vi "ROI entry-Set ROI tool on Clear All.vi"(8 "error in (no error)":errorcluster, 11 "Last ROI ID Enum":T1) -> (0 "error out":errorcluster)   [LabVIEW 2013]
uses:
  Typedefs/ROI ID Enum.ctl
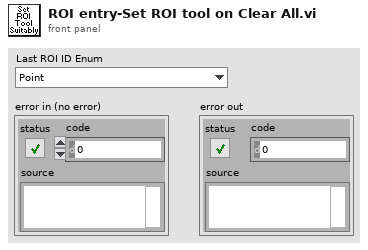
[diagram p1: front panel]
types:
  T1 = typedef "ROI ID Enum.ctl" = enum16{"Point", "MiniScan", "Comp. MiniScan", "Rectangle", "Comp. volume", "Arb. plane point"}
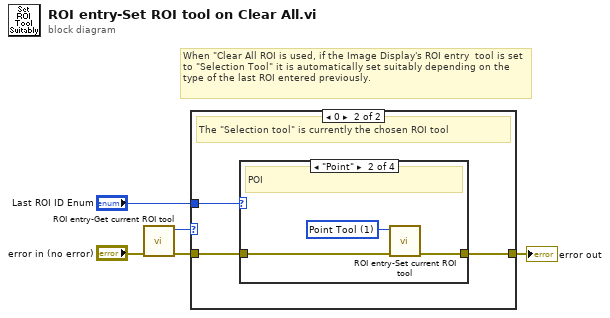
[diagram p0: block diagram]
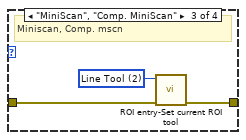
[diagram p4: hidden frame]
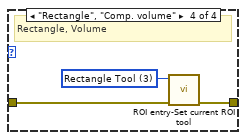
[diagram p5: hidden frame]
diagram:
  # "When \"Clear All ROI is used, if the Image Display's ROI entry  tool is set to \"Selection Tool\" it is automatically set suitably depending on the type of the last ROI entered previously."
  n1 = call "ROI entry-Get current ROI tool.vi"("error in (no error)"="error in (no error)") -> ("error out"=w3:errorcluster, "Current ROI Tool"=w2:u32)  [unwired: 9 in]
  n2 = case shown="0" w2 {
    tunnel: [w6 w9] -> w5
    tunnel: w3 -> [w6 w7]
    tunnel: "Last ROI ID Enum" -> [_ w8]
    frame Default {
      # "The chosen ROI tool is not the \"Selection tool\"."
    }
    frame 0 {
      # "The \"Selection tool\" is currently the chosen ROI tool"
      n3 = case shown="\"Point\"" w8 {
        tunnel: w7 -> [w10 w12 w15 w19]
        tunnel: [w10 w11 w14 w18] -> w9
        frame Default {
          # "Invalid"
        }
        frame "Point" {
          w13 = u32 1 items=["Zoom Tool"=8, "Selection Tool"=0, "Pan Tool"=9, "Point Tool"=1, "Line Tool"=2, "Rectangle Tool"=3, "Rotated Rectangle Tool"=12, "Polyline Tool"=10, "Polygon Tool"=5, "Freehand Tool"=11, "Closed Freehand Tool"=6, "Ellipse Tool"=4, "Annulus Tool"=7] ("Current ROI Tool")
          # "POI"
          n4 = call "ROI entry-Set current ROI tool.vi"("error in (no error)"=w12, "Current ROI Tool"=w13) -> ("error out"=w11:errorcluster)  [unwired: 9 in]
        }
        frame "MiniScan", "Comp. MiniScan" {
          w16 = u32 2 items=["Zoom Tool"=8, "Selection Tool"=0, "Pan Tool"=9, "Point Tool"=1, "Line Tool"=2, "Rectangle Tool"=3, "Rotated Rectangle Tool"=12, "Polyline Tool"=10, "Polygon Tool"=5, "Freehand Tool"=11, "Closed Freehand Tool"=6, "Ellipse Tool"=4, "Annulus Tool"=7] ("Current ROI Tool")
          # "Miniscan, Comp. mscn"
          n5 = call "ROI entry-Set current ROI tool.vi"("error in (no error)"=w15, "Current ROI Tool"=w16) -> ("error out"=w14:errorcluster)  [unwired: 9 in]
        }
        frame "Rectangle", "Comp. volume" {
          w17 = u32 3 items=["Zoom Tool"=8, "Selection Tool"=0, "Pan Tool"=9, "Point Tool"=1, "Line Tool"=2, "Rectangle Tool"=3, "Rotated Rectangle Tool"=12, "Polyline Tool"=10, "Polygon Tool"=5, "Freehand Tool"=11, "Closed Freehand Tool"=6, "Ellipse Tool"=4, "Annulus Tool"=7] ("Current ROI Tool")
          # "Rectangle, Volume"
          n6 = call "ROI entry-Set current ROI tool.vi"("error in (no error)"=w19, "Current ROI Tool"=w17) -> ("error out"=w18:errorcluster)  [unwired: 9 in]
        }
      }
    }
  }
  "error out" <- w5
